vi "ROSNode.vi"(2 "Response":T1, 3 "ROS":T3={"topic port"=7000, "Node"="/LVROS", "topic"="/LVROS", "type"="", "node port"=7000, "error "={"status"=FALSE, "code"=0, "source"=""}, "Direction"=enum."Node", "Update (ms)"=1, "FIFO size"=1}) -> ()   [LabVIEW 2012]
doc: "Performs the functions of a ROS node: adds a publisher to the registered publisher list and registers with the master, starts and updates publishers, adds subscribers, and opens ports for subscribers and publishers"
uses:
  <userlib>/ROSforLV/ROS/Code/SubVIs/_ROSControl.ctl
  <userlib>/ROSforLV/ROS/Code/SubVIs/_ROSDirection.ctl
  <userlib>/ROSforLV/ROS/Code/Console/Servers/ServerSubs/MyState.ctl
  <userlib>/ROSforLV/ROS/Code/Console/Servers/ServerSubs/ROSLog.ctl
  <vilib>/Utility/miscctls.llb/LVPointTypeDef.ctl
  <userlib>/ROSforLV/ROS/Code/_ROSDefinition.vi
  <vilib>/Platform/browser.llb/Open URL in Default Browser (string).vi
panel:
  out "Color Code":picture
  out "Status out":T2[](array[typedef])
  out "Status":string
  out "Connections":bool
  out "Boundaries":cluster{i32, i32}[](array[cluster])=[{10, 22}, {30, 42}, {50, 62}]
  out "selection":i32=-1
  in  "HTML":bool
  out "ROS Master":string="130.64.16.138:11311"
  out "Registered":T3[](array[typedef])
  out "Last requestTopic":string
  out "Subscribers":T5(array[cluster])
  out "Queue log":string
  out "MyState":T2
  out "Setup":string
  in  "stop":bool
  out "HTML":picture
  out "Servers":picture
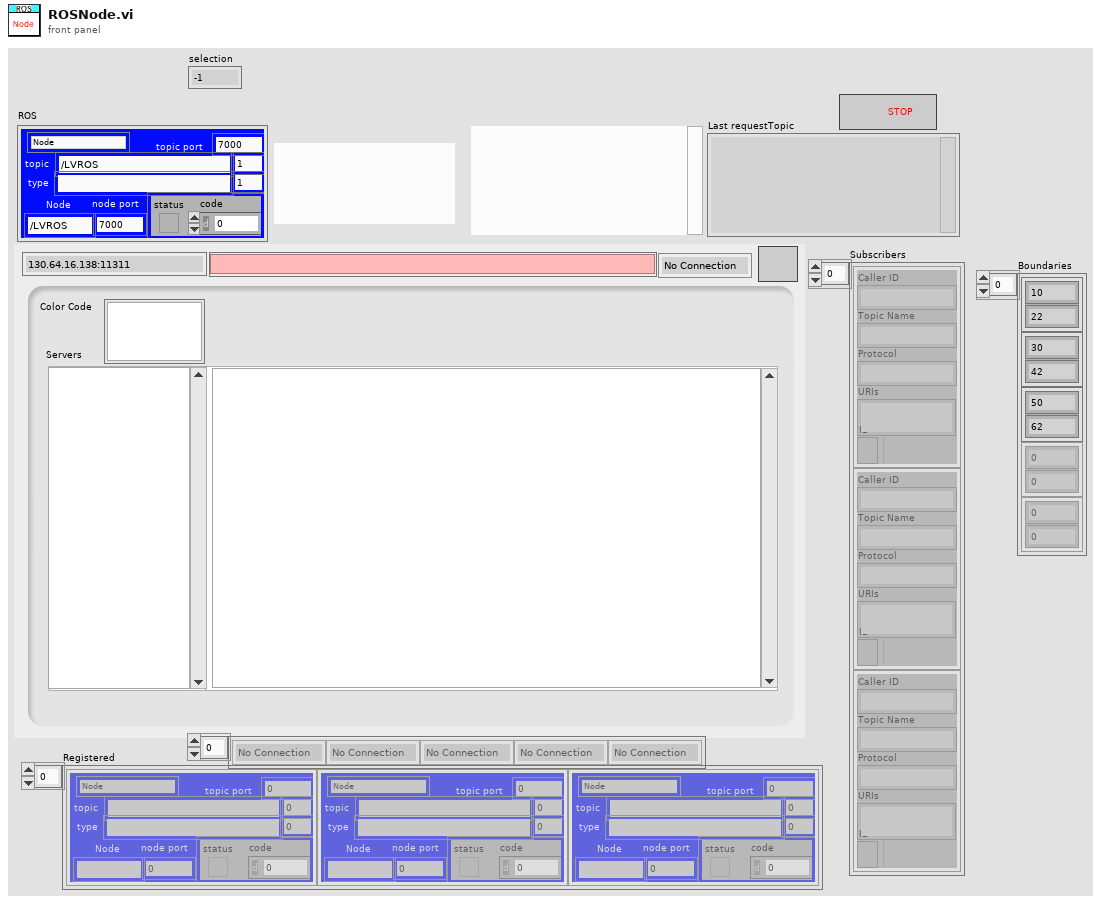
[diagram p1: front panel]
types:
  T1 = cluster{"Code":i32, "Status Message":string, "Nodes with this topic":string[]}
  T2 = typedef "MyState.ctl" = enum16{"No Connection", "Registered", "Connected", "Close"}
  T3 = typedef "_ROSControl.ctl" = cluster{"topic port":u16, "Node":string, "topic":string, "type":string, "node port":u16, "error ":errorcluster, "Direction":T4, "Update (ms)":u16, "FIFO size":u16}
  T4 = typedef "_ROSDirection.ctl" = enum16{"Node", "Publisher", "Subscriber", "ServiceClient", "ServiceProvider"}
  T5 = cluster{"Caller ID":string, "Topic Name":string, "Protocol":string, "URIs":string, "ID":refnum<k5>}[]
  T6 = enum16{"Reset Log", "Add Client", "Remove Client", "Add Task"}
  T7 = typedef "ROSLog.ctl" = cluster{"Sent":string, "Reply":string, "MethodName":string, "success":bool, "Dir1":string, "Dir2":string, "Time Stamp":string, "error":errorcluster, "Preamble":string, "Midamble":string, "Postamble":string}
  T8 = cluster{"Caller ID":string, "Topic Name":string, "Protocol":string, "URI":string, "ID":refnum<k5>}
  T9 = cluster{"Caller ID":string, "Topic Name":string, "Protocol":string, "URI":string, "ID":refnum<k5>}[]
  T10 = typedef "LVPointTypeDef.ctl" = cluster{"Horizontal":i16, "Vertical":i16}
  T11 = typedef "LVMouseTypeDef.ctl" = cluster{"Mouse Position":cluster{"X":i32, "Y":i32}, "Mouse Modifiers":cluster{"Button Down":bool, "Shift Mod":bool, "Menu Mod":bool, "Option Mod":bool}}
  T12 = cluster{"Caller ID":string, "Topic Name":string, "Node URIs":string[]}
  T13 = enum32{"Invalid", "Standard", "Closed", "Hidden", "Minimized", "Maximized"}
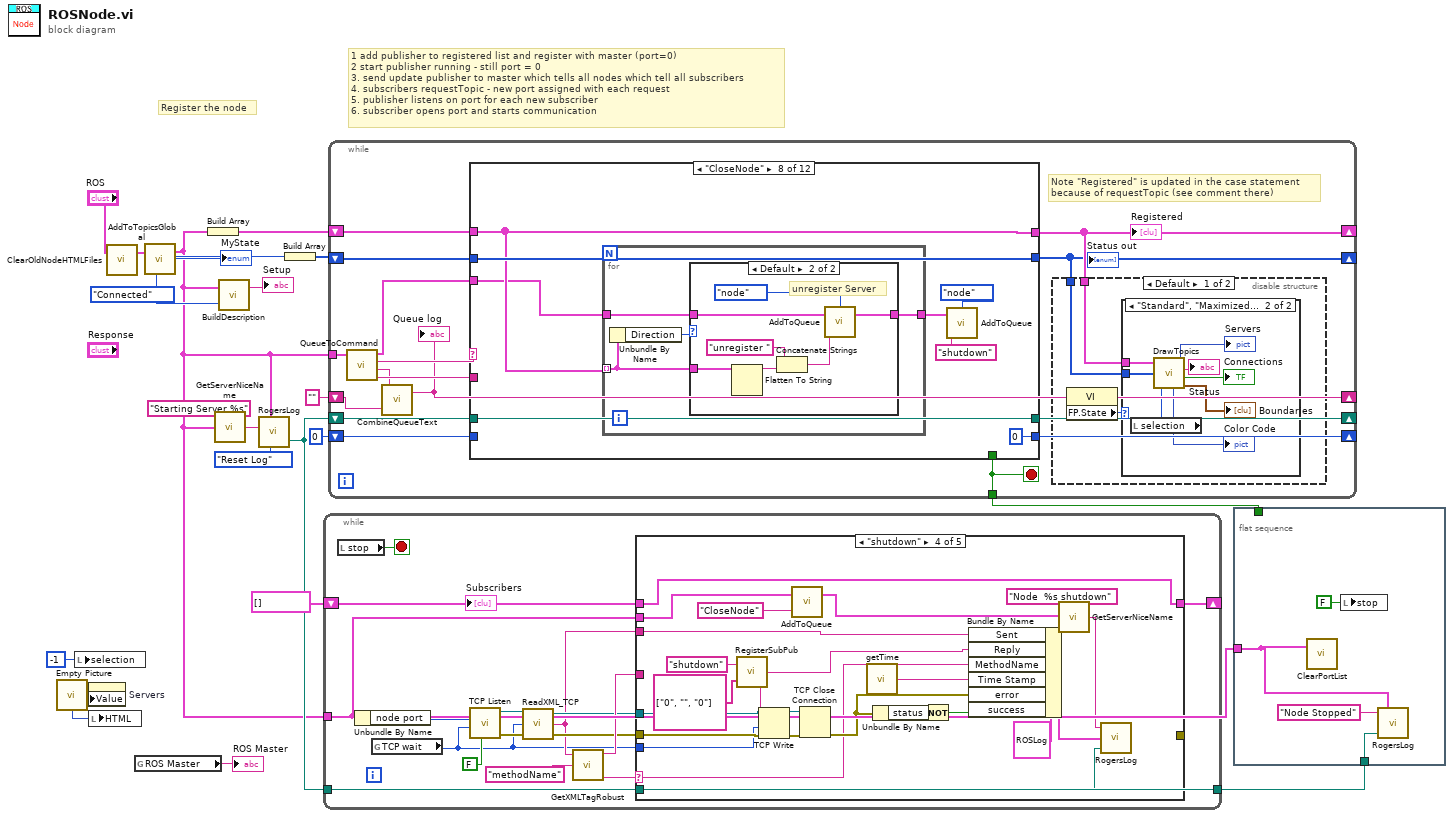
[diagram p0: block diagram]
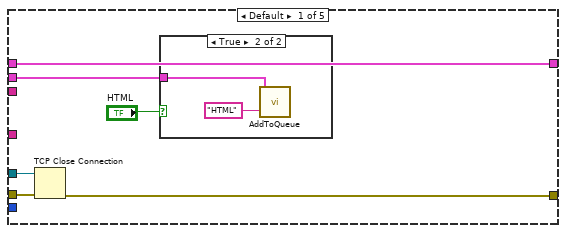
[diagram p2: hidden frame]
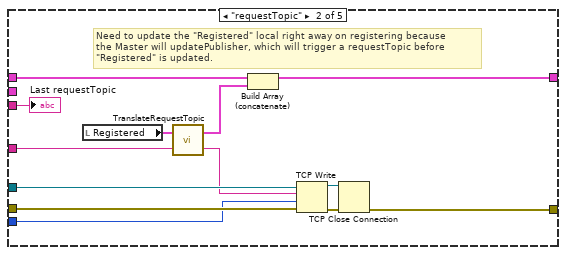
[diagram p4: hidden frame]
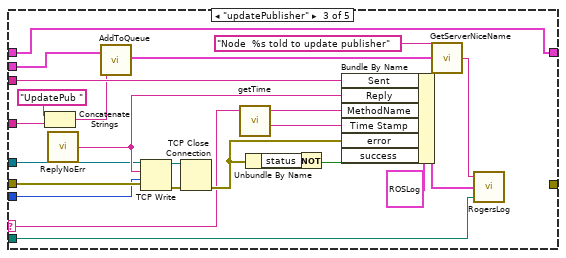
[diagram p5: hidden frame]
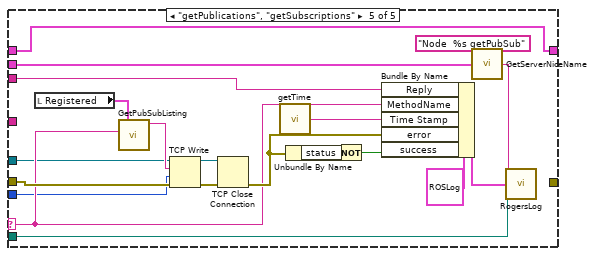
[diagram p6: hidden frame]
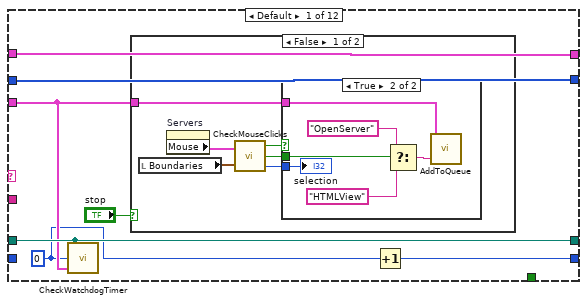
[diagram p9: hidden frame]
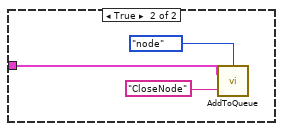
[diagram p11: hidden frame]
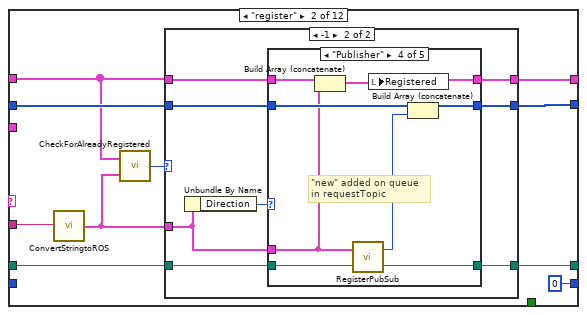
[diagram p12: hidden frame]
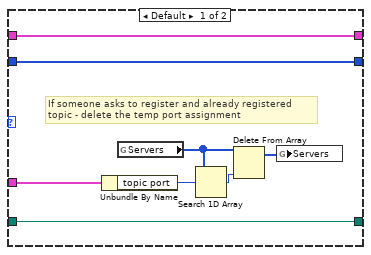
[diagram p13: hidden frame]
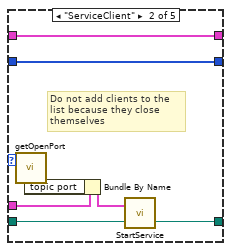
[diagram p15: hidden frame]
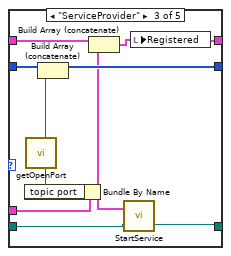
[diagram p16: hidden frame]
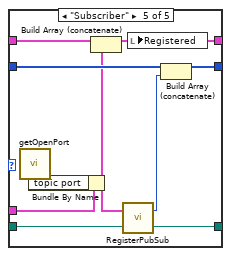
[diagram p17: hidden frame]
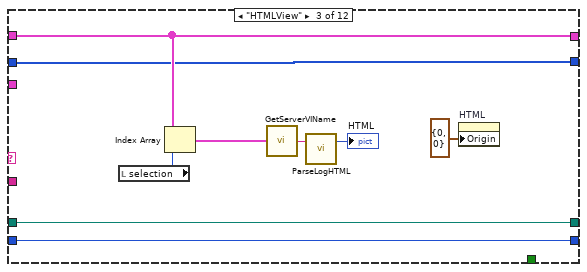
[diagram p18: hidden frame]
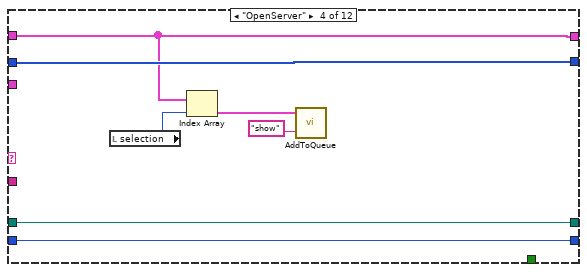
[diagram p19: hidden frame]
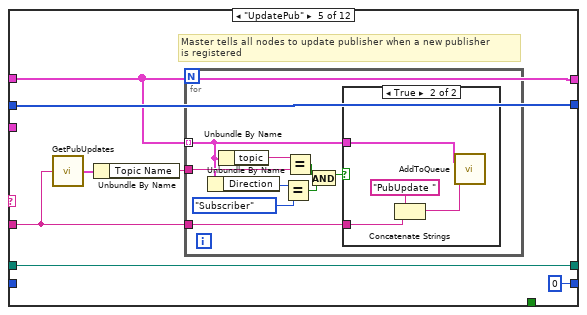
[diagram p20: hidden frame]
diagram:
  w12 = MyState."Connected" ("MyState")
  # "Register the node"
  # "1 add publisher to registered list and register with master (port=0)\n2 start publisher running - still port = 0\n3. send update publisher to master which tells all nodes which tell all subscribers\n4. subscribers requestTopic - new port assigned with each request\n5. publisher listens on port for each new subscriber\n6. subscriber opens port and starts communication"
  n1 = call "Empty Picture"() -> ("empty picture"=w10:picture)
  n2 = local write "selection"(-1 ("selection")) -> ()
  n3 = property on="Servers" class="Pict"("Value"=w10) -> ()  [unwired: 2 in, 2 out]
  n4 = local write "HTML"(w10) -> ()
  n5 = call <userlib>:"ClearOldNodeHTMLFiles.vi"("ROS"="ROS") -> ("ROS out"=w2:T3)  [unwired: 2 in]
  n6 = global read "_ROSDefinition.vi" "ROS Master"() -> (→"ROS Master":string)
  n7 = call <userlib>:"AddToTopicsGlobal.vi"("ROS in"=w2) -> ("ROS out"=w1:T3)  [unwired: 2 in]
  n8 = Build Array(w1) -> (w13:T3[])
  n9 = call <userlib>:"GetServerNiceName.vi"("ROS"=w1, "Text to add"="Starting Server %s") -> ("String"=w17:string)
  n10 = call <userlib>:"BuildDescription.vi"("MyState"=w12, "ROS in"=w1) -> ("Setup"=→"Setup":string)  [unwired: 1 in]
  n11 = call <userlib>:"RogersLog.vi"("Text to add"=w17, "ROS"=w1, "Task"=T6."Reset Log") -> ("LogPath out"=w7:path)  [unwired: 2 in, 1 out]
  n12 = Build Array(w12) -> (w11:T2[])
  n13 = while {
    shift-right: [w26] -> _
    shift-left: T5 [] ("Subscribers") -> [w27]
    tunnel: w1 -> [w21]
    tunnel: w7 -> [w20]
    tunnel: [w20] -> w4
    stop <- w35 stop-if-true
    n14 = local read "stop"() -> (w35:bool)
    n15 = Unbundle By Name(w21) -> ("node port"=w31:u16)
    n16 = global read "_ROSDefinition.vi" "TCP wait"() -> (w22:i32)
    n17 = call <vilib>:"TCP Listen.vi"("resolve remote address (T)"=FALSE, "timeout ms (wait forever: -1)"=w22, "port"=w31) -> ("error out"=w33:errorcluster, "connection ID"=w32:refnum<k5>)  [unwired: 4 in, 3 out]
    n18 = call <userlib>:"ReadXML_TCP.vi"("error in"=w33, "timeout ms (3000)"=w22, "connection ID in"=w32) -> ("error out"=w24:errorcluster, "data out"=w23:string, "connection ID out"=w25:refnum<k5>)
    n19 = call <userlib>:"GetXMLTagRobust.vi"("Tag"="methodName", "String"=w23) -> ("value"=w29:string, "String w/o Tag"=w28:string)  [unwired: 1 in, 2 out]
    n20 = case shown="\"shutdown\"" w29 {
      selector: w29 -> [_ _ w68 w97 w108]
      tunnel: w28 -> [_ w48 w65 _ _]
      tunnel: w27 -> [w41 w56 w66 w96 w115]
      tunnel: [w41 w55 w66 w96 w115] -> w26
      tunnel: w25 -> [w37 w52 w70 w86 w104]
      tunnel: w24 -> [w38 w51 w69 w88 w110]
      tunnel: w23 -> [_ w50 w71 w91 w116]
      tunnel: w22 -> [_ w45 w67 w83 w105]
      tunnel: w21 -> [w40 _ w57 w82 w109]
      tunnel: w20 -> [_ _ w60 w92 w111]
      tunnel: [w36 w44 _ _ _] -> _
      frame Default {
        n21 = TCP Close Connection(connection ID=w37, error in (no error)=w38) -> (error out=w36:errorcluster)  [unwired: 1 in, 1 out]
        n22 = case shown="True" "HTML" {
          tunnel: w40 -> [_ w42]
          frame False {
          }
          frame True {
            n23 = call <userlib>:"AddToQueue.vi"("Cmd"="HTML" ("element"), "ROS"=w42) -> ()  [unwired: 3 in, 1 out]
          }
        }
      }
      frame "requestTopic" {
        # "Need to update the \"Registered\" local right away on registering because\nthe Master will updatePublisher, which will trigger a requestTopic before\n\"Registered\" is updated."
        n24 = local read "Registered"() -> (w49:T3[])
        n25 = call <userlib>:"TranslateRequestTopic.vi"("String w/o Tag"=w48, "Registered"=w49) -> ("XML"=w47:string, "New Sub"=w46:T8)
        n26 = Build Array (concatenate)(w56, w46) -> (w55:T9)
        n27 = TCP Write(connection ID=w52, data in=w47, error in (no error)=w51, 9:w45) -> (connection ID out=w54:refnum<k5>, error out=w53:errorcluster)  [unwired: 1 out]
        n28 = TCP Close Connection(connection ID=w54, error in (no error)=w53) -> (error out=w44:errorcluster)  [unwired: 1 in, 1 out]
        "Last requestTopic" <- w50
      }
      frame "updatePublisher" {
        n29 = Concatenate Strings("UpdatePub " ("string"), w65) -> (w58:string)
        n30 = call <userlib>:"ReplyNoErr.vi"() -> ("msg out"=w75:string)  [unwired: 1 in]
        n31 = call <userlib>:"AddToQueue.vi"("Cmd"=w58, "ROS"=w57) -> ("ROS out"=w59:T3)  [unwired: 3 in]
        n32 = TCP Write(connection ID=w70, data in=w75, error in (no error)=w69, 9:w67) -> (connection ID out=w77:refnum<k5>, error out=w76:errorcluster)  [unwired: 1 out]
        n33 = TCP Close Connection(connection ID=w77, error in (no error)=w76) -> (error out=w74:errorcluster)  [unwired: 1 in, 1 out]
        n34 = call <userlib>:"getTime.vi"() -> ("Current Time"=w78:string)  [unwired: 1 in]
        n35 = Unbundle By Name(w74) -> ("status"=w73:bool)
        n36 = Not(x=w73) -> (.not. x?=w72:bool)
        n37 = Bundle By Name(cluster=T7 {"Sent"="", "Reply"="", "MethodName"="", "success"=TRUE, "Dir1"="From Master", "Dir2"="To Master", "Time Stamp"="", "error"={"status"=FALSE, "code"=0, "source"=""}, "Preamble"="", "Midamble"="", "Postamble"=""} ("Log"), "Sent"=w71, "Reply"=w75, "MethodName"=w68, "Time Stamp"=w78, "error"=w74, "success"=w72) -> (w63:T7)
        n38 = call <userlib>:"GetServerNiceName.vi"("ROS"=w59, "Text to add"="Node  %s told to update publisher") -> ("String"=w61:string)
        n39 = call <userlib>:"RogersLog.vi"("Text to add"=w61, "Log"=w63, "LogPath in"=w60) -> ()  [unwired: 2 in, 2 out]
      }
      frame "shutdown" {
        n40 = call <userlib>:"RegisterSubPub.vi"("Parameters"=string[] ["0", "", "0"], "MethodName"="shutdown") -> ("XML"=w85:string)
        n41 = TCP Write(connection ID=w86, data in=w85, error in (no error)=w88, 9:w83) -> (connection ID out=w84:refnum<k5>, error out=w87:errorcluster)  [unwired: 1 out]
        n42 = call <userlib>:"AddToQueue.vi"("Cmd"="CloseNode" ("element"), "ROS"=w82) -> ("ROS out"=w80:T3)  [unwired: 3 in]
        n43 = TCP Close Connection(connection ID=w84, error in (no error)=w87) -> (error out=w100:errorcluster)  [unwired: 1 in, 1 out]
        n44 = call <userlib>:"getTime.vi"() -> ("Current Time"=w101:string)  [unwired: 1 in]
        n45 = Unbundle By Name(w100) -> ("status"=w99:bool)
        n46 = Not(x=w99) -> (.not. x?=w98:bool)
        n47 = Bundle By Name(cluster=T7 {"Sent"="", "Reply"="", "MethodName"="", "success"=TRUE, "Dir1"="From Master", "Dir2"="To Master", "Time Stamp"="", "error"={"status"=FALSE, "code"=0, "source"=""}, "Preamble"="", "Midamble"="", "Postamble"=""} ("Log"), "Sent"=w91, "Reply"=w85, "MethodName"=w97, "Time Stamp"=w101, "error"=w100, "success"=w98) -> (w95:T7)
        n48 = call <userlib>:"GetServerNiceName.vi"("ROS"=w80, "Text to add"="Node  %s shutdown") -> ("String"=w93:string)
        n49 = call <userlib>:"RogersLog.vi"("Text to add"=w93, "Log"=w95, "LogPath in"=w92) -> ()  [unwired: 2 in, 2 out]
      }
      frame "getPublications", "getSubscriptions" {
        n50 = local read "Registered"() -> (w106:T3[])
        n51 = call <userlib>:"GetPubSubListing.vi"("Method"=w108, "Registered"=w106) -> ("StatusMessage"=w107:string)  [unwired: 9 in]
        n52 = TCP Write(connection ID=w104, data in=w107, 9:w105) -> (connection ID out=w103:refnum<k5>)  [unwired: 1 in, 2 out]
        n53 = TCP Close Connection(connection ID=w103, error in (no error)=w110) -> (error out=w119:errorcluster)  [unwired: 1 in, 1 out]
        n54 = call <userlib>:"getTime.vi"() -> ("Current Time"=w120:string)  [unwired: 1 in]
        n55 = Unbundle By Name(w119) -> ("status"=w118:bool)
        n56 = Not(x=w118) -> (.not. x?=w117:bool)
        n57 = Bundle By Name(cluster=T7 {"Sent"="", "Reply"="", "MethodName"="", "success"=TRUE, "Dir1"="From Master", "Dir2"="To Master", "Time Stamp"="", "error"={"status"=FALSE, "code"=0, "source"=""}, "Preamble"="", "Midamble"="", "Postamble"=""} ("Log"), "Reply"=w116, "MethodName"=w108, "Time Stamp"=w120, "error"=w119, "success"=w117) -> (w114:T7)
        n58 = call <userlib>:"GetServerNiceName.vi"("ROS"=w109, "Text to add"="Node  %s getPubSub") -> ("String"=w112:string)
        n59 = call <userlib>:"RogersLog.vi"("Text to add"=w112, "Log"=w114, "LogPath in"=w111) -> ()  [unwired: 2 in, 2 out]
      }
    }
    "Subscribers" <- w27
  }
  n60 = while {
    tunnel: w1 -> [w131]
    tunnel: [w134] -> w14
    shift-right: [w130] -> _
    shift-left: w13 -> [w135]
    shift-right: [w132] -> _
    shift-left: w7 -> [w133]
    shift-right: [w128] -> _
    shift-left: w11 -> [w129]
    shift-right: [w126] -> _
    shift-left: 0 ("selection") -> [w127]
    shift-right: [w125] -> _
    shift-left: "" ("New List") -> [w124]
    stop <- w134 stop-if-true
    # "Note \"Registered\" is updated in the case statement\nbecause of requestTopic (see comment there)"
    n61 = call <userlib>:"QueueToCommand.vi"("ROS"=w131) -> ("ROS out"=w122:T3, "Command"=w137:string, "Queue log"=w123:string, "data"=w136:string)  [unwired: 2 in]
    n62 = call <userlib>:"CombineQueueText.vi"("Old List"=w124, "Queue In"=w123) -> ("New List"=w125:string)  [unwired: 1 in]
    "Queue log" <- w125
    n63 = case shown="\"CloseNode\"" w137 {
      tunnel: w136 -> [_ w180 _ _ w251 w279 _ _ _ _ w337 _]
      tunnel: [w154 w179 w237 w247 w252 w273 w299 w307 w327 w331 w340 w357] -> w130
      tunnel: w135 -> [w154 w173 w237 w247 w252 w274 w300 w307 w327 w331 w340 w357]
      tunnel: [_ _ _ _ _ _ _ _ w324 _ _ _] -> w134
      tunnel: w133 -> [w152 w178 w239 w249 w256 w278 w302 w309 w325 w330 w346 w355]
      tunnel: [w152 w177 w239 w249 w256 w277 w302 w309 w325 w330 w346 w355] -> w132
      tunnel: w122 -> [w151 _ _ _ _ _ w294 w306 _ _ _ _]
      tunnel: w129 -> [w153 w176 w235 w248 w255 w272 w298 w310 w326 w329 w343 w356]
      tunnel: [w153 w175 w235 w248 w255 w271 w297 w310 w326 w329 w342 w356] -> w128
      tunnel: w127 -> [_ _ w234 w245 _ _ _ _ w323 w328 _ w354]
      tunnel: [w150 0 w234 w245 0 0 0 0 w323 w328 0 ("selection") w354] -> w126
      frame Default {
        w149 = 0 ("selection")
        n64 = call <userlib>:"CheckWatchdogTimer.vi"("ROS"=w151, "itteration"=w149, "LogPath in"=w152) -> ()  [unwired: 3 in]
        n65 = case shown="False" "stop" {
          tunnel: w151 -> [w158 w169]
          frame False {
            n66 = local read "Boundaries"() -> (w157:cluster{i32, i32}[])
            n67 = property on="Servers" class="Pict"() -> ("Mouse"=w159:T11)  [unwired: 2 in, 2 out]
            n68 = call <userlib>:"CheckMouseClicks.vi"("Mouse"=w159, "Boundaries"=w157) -> ("Change?"=w160:bool, "Shift?"=w156:bool, "selection"=w161:i32)
            n69 = case shown="True" w160 {
              tunnel: w161 -> [_ w167]
              tunnel: w158 -> [_ w162]
              tunnel: w156 -> [_ w165]
              frame False {
              }
              frame True {
                n70 = Select(t="OpenServer" ("element"), s=w165, f="HTMLView" ("element")) -> (s? t:f=w163:string)
                n71 = call <userlib>:"AddToQueue.vi"("Cmd"=w163, "ROS"=w162) -> ()  [unwired: 3 in, 1 out]
                "selection" <- w167
              }
            }
          }
          frame True {
            n72 = call <userlib>:"AddToQueue.vi"("Cmd"="CloseNode" ("element"), "ROS"=w169, "Type"=enum16{"topic", "node"}."node" ("Name")) -> ()  [unwired: 2 in, 1 out]
          }
        }
        n73 = Increment(x=w149) -> (x+1=w150:i32)
      }
      frame "register" {
        n74 = call <userlib>:"ConvertStringtoROS.vi"("string in"=w180) -> ("ROS"=w172:T3)
        n75 = call <userlib>:"CheckForAlreadyRegistered.vi"("ROS"=w172, "Registered"=w173) -> ("index of element"=w174:i32)
        n76 = case shown="-1" w174 {
          tunnel: w172 -> [w185 w189]
          tunnel: [w188 w196] -> w179
          tunnel: w173 -> [w188 w195]
          tunnel: w178 -> [w186 w194]
          tunnel: [w186 w193] -> w177
          tunnel: w176 -> [w187 w192]
          tunnel: [w187 w191] -> w175
          frame Default {
            # "If someone asks to register and already registered\ntopic - delete the temp port assignment"
            n77 = Unbundle By Name(w185) -> ("topic port"=w184:u16)
            n78 = global read "_ROSDefinition.vi" "Servers"() -> (w182:u16[])
            n79 = Search 1D Array(1D array=w182, element=w184) -> (index of element=w183:i32)  [unwired: 1 in]
            n80 = Delete From Array(array=w182, index=w183) -> (array with subset deleted=w181:u16[])  [unwired: 1 in, 1 out]
            n81 = global write "_ROSDefinition.vi" "Servers"(w181) -> ()
          }
          frame -1 {
            n82 = Unbundle By Name(w189) -> ("Direction"=w190:T4)
            n83 = case shown="\"Publisher\"" w190 {
              tunnel: [w199 w201 w212 w216 w224] -> w196
              tunnel: w195 -> [w199 w201 w214 w223 w233]
              tunnel: w194 -> [w197 w206 w208 w222 w232]
              tunnel: [w197 w205 w207 w221 w231] -> w193
              tunnel: w192 -> [w198 w200 w213 w220 w230]
              tunnel: [w198 w200 w211 w219 w229] -> w191
              tunnel: w189 -> [_ w203 w215 w217 w226]
              frame "Node", Default {
              }
              frame "ServiceClient" {
                # "Do not add clients to the \nlist because they close \nthemselves"
                n84 = call <userlib>:"getOpenPort.vi"() -> ("port"=w204:u16)
                n85 = Bundle By Name(cluster=w203, "topic port"=w204) -> (w202:T3)
                n86 = call <userlib>:"StartService.vi"("LogPath in"=w206, "New server ROS"=w202) -> ("LogPath out"=w205:path)  [unwired: 1 out]
              }
              frame "ServiceProvider" {
                n87 = call <userlib>:"getOpenPort.vi"() -> ("port"=w210:u16)
                n88 = Bundle By Name(cluster=w215, "topic port"=w210) -> (w209:T3)
                n89 = Build Array (concatenate)(w213, w210) -> (w211:u16[])
                n90 = Build Array (concatenate)(w214, w209) -> (w212:T3[])
                n91 = call <userlib>:"StartService.vi"("LogPath in"=w208, "New server ROS"=w209) -> ("LogPath out"=w207:path)  [unwired: 1 out]
                n92 = local write "Registered"(w212) -> ()
              }
              frame "Publisher" {
                # "\"new\" added on queue\nin requestTopic"
                n93 = Build Array (concatenate)(w223, w217) -> (w216:T3[])
                n94 = call <userlib>:"RegisterPubSub.vi"("LogPath in"=w222, "New server ROS"=w217) -> ("LogPath out"=w221:path, "MyState"=w218:T2)
                n95 = local write "Registered"(w216) -> ()
                n96 = Build Array (concatenate)(w220, w218) -> (w219:u16[])
              }
              frame "Subscriber" {
                n97 = call <userlib>:"getOpenPort.vi"() -> ("port"=w227:u16)
                n98 = Bundle By Name(cluster=w226, "topic port"=w227) -> (w225:T3)
                n99 = Build Array (concatenate)(w233, w225) -> (w224:T3[])
                n100 = call <userlib>:"RegisterPubSub.vi"("LogPath in"=w232, "New server ROS"=w225) -> ("LogPath out"=w231:path, "MyState"=w228:T2)
                n101 = local write "Registered"(w224) -> ()
                n102 = Build Array (concatenate)(w230, w228) -> (w229:u16[])
              }
            }
          }
        }
      }
      frame "HTMLView" {
        n103 = local read "selection"() -> (w240:i32)
        n104 = Index Array(array=w237, index=w240) -> (element=w236:T3)
        n105 = call <userlib>:"GetServerVIName.vi"("ROS"=w236) -> ("vi name"=w241:string)
        n106 = call <userlib>:"ParseLogHTML.vi"("vi name"=w241) -> ("2D Picture"=→"HTML":picture)  [unwired: 1 in, 1 out]
        n107 = property on="HTML" class="Pict"("Origin"=T10 {"Horizontal"=0, "Vertical"=0}) -> ()  [unwired: 2 in, 2 out]
      }
      frame "OpenServer" {
        n108 = local read "selection"() -> (w246:i32)
        n109 = Index Array(array=w247, index=w246) -> (element=w244:T3)
        n110 = call <userlib>:"AddToQueue.vi"("Cmd"="show" ("element"), "ROS"=w244) -> ()  [unwired: 3 in, 1 out]
      }
      frame "UpdatePub" {
        # "Master tells all nodes to update publisher when a new publisher\nis registered"
        n111 = call <userlib>:"GetPubUpdates.vi"("XML"=w251) -> ("PubUpdate"=w254:T12)
        n112 = Unbundle By Name(w254) -> ("Topic Name"=w253:string)
        n113 = for {
          tunnel: w252 -> [w258] mode=indexing
          tunnel: w253 -> [w264]
          tunnel: w251 -> [w257]
          n114 = Unbundle By Name(w258) -> ("Direction"=w263:T4)
          n115 = Unbundle By Name(w258) -> ("topic"=w265:string)
          n116 = Equal?(x=w263, y=_ROSDirection."Subscriber" ("Direction")) -> (x = y?=w260:bool)
          n117 = Equal?(x=w265, y=w264) -> (x = y?=w261:bool)
          n118 = And(x=w261, y=w260) -> (x .and. y?=w259:bool)
          n119 = case shown="True" w259 {
            tunnel: w258 -> [_ w266]
            tunnel: w257 -> [_ w268]
            frame False {
            }
            frame True {
              n120 = Concatenate Strings("PubUpdate " ("string"), w268) -> (w267:string)
              n121 = call <userlib>:"AddToQueue.vi"("Cmd"=w267, "ROS"=w266) -> ()  [unwired: 3 in, 1 out]
            }
          }
        }
      }
      frame "unregister" {
        n122 = call <userlib>:"ConvertStringtoROS.vi"("string in"=w279) -> ("ROS"=w276:T3)
        n123 = call <userlib>:"CheckForAlreadyRegistered.vi"("ROS"=w276, "Registered"=w274) -> ("index of element"=w275:i32)
        n124 = case shown="Default" w275 {
          selector: w275 -> [_ w286]
          tunnel: w278 -> [w280 w292]
          tunnel: [w280 w291] -> w277
          tunnel: w276 -> [_ w284]
          tunnel: w274 -> [w282 w285]
          tunnel: [w282 w289] -> w273
          tunnel: w272 -> [w281 w288]
          tunnel: [w281 w287] -> w271
          frame -1 {
          }
          frame Default {
            # "Stop Server"
            n125 = Delete From Array(array=w285, index=w286) -> (array with subset deleted=w289:T3[])  [unwired: 1 in, 1 out]
            n126 = Delete From Array(array=w288, index=w286) -> (array with subset deleted=w287:u16[])  [unwired: 1 in, 1 out]
            n127 = call <userlib>:"UnRegisterPubSub.vi"("LogPath in"=w292, "ROS"=w284) -> ("LogPath out"=w291:path)  [unwired: 1 out]
            n128 = call <userlib>:"AddToQueue.vi"("Cmd"="done" ("element"), "ROS"=w284, "Type"=enum16{"topic", "node"}."topic" ("Name")) -> ()  [unwired: 2 in, 1 out]
          }
        }
      }
      frame "shutdown" {
        # "Stop Server"
        n129 = call <userlib>:"CheckForAlreadyRegistered.vi"("ROS"=w294, "Registered"=w300) -> ("index of element"=w301:i32)
        n130 = call <userlib>:"AddToQueue.vi"("Cmd"="done" ("element"), "ROS"=w294, "Type"=enum16{"topic", "node"}."node" ("Name")) -> ()  [unwired: 2 in, 1 out]
        n131 = Delete From Array(array=w300, index=w301) -> (array with subset deleted=w299:T3[])  [unwired: 1 in, 1 out]
        n132 = Delete From Array(array=w298, index=w301) -> (array with subset deleted=w297:u16[])  [unwired: 1 in, 1 out]
      }
      frame "CloseNode" {
        n133 = for {
          tunnel: w307 -> [w314] mode=indexing
          tunnel: w306 -> [w312]
          tunnel: [w311] -> w304
          n134 = Unbundle By Name(w314) -> ("Direction"=w313:T4)
          n135 = case shown="Default" w313 {
            tunnel: w314 -> [_ w322]
            tunnel: w312 -> [w315 w319]
            tunnel: [w315 w316] -> w311
            frame "Node" {
              # "Provider closes in server\nand Node closes in \nshutdown."
            }
            frame Default {
              # "unregister Server"
              n136 = Flatten To String(anything=w322) -> (data string=w321:string)  [unwired: 3 in, 2 out]
              n137 = Concatenate Strings("unregister " ("element"), w321) -> (w318:string)
              n138 = call <userlib>:"AddToQueue.vi"("Cmd"=w318, "ROS"=w319, "Type"=enum16{"topic", "node"}."node" ("Name")) -> ("ROS out"=w316:T3)  [unwired: 2 in]
            }
          }
        }
        n139 = call <userlib>:"AddToQueue.vi"("Cmd"="shutdown" ("element"), "ROS"=w304, "Type"=enum16{"topic", "node"}."node" ("Name")) -> ()  [unwired: 2 in, 1 out]
      }
      frame "done" {
        w324 = TRUE ("stop")
        n140 = local write "stop"(w324) -> ()
      }
      frame "HTML" {
        n141 = disable-structure shown="Default" {
          disable-tunnel: w330 -> [w332 _]
          frame condition #0 (active) {
            n142 = call <userlib>:"GetLogFilePath.vi"() -> ("LogFolder"=w334:path)  [unwired: 2 in, 1 out]
            n143 = Build Path(base path=w334, name or relative path="index.html" ("pattern")) -> ()  [unwired: 1 out]
            n144 = call <vilib>:"Path to URL.vi"("path"=w332) -> ("url"=w335:string)
            n145 = call-poly <vilib>:"Open URL in Default Browser.vi"("URL"=w335) -> ()  [unwired: 5 in, 2 out]
          }
          frame condition #1 {
          }
        }
      }
      frame "status" {
        n146 = Match Pattern(string=w337, regular expression="STATE") -> (before substring=w341:string, after substring=w344:string)  [unwired: 1 in, 2 out]
        n147 = call <userlib>:"ConvertStringtoROS.vi"("string in"=w341) -> ("ROS"=w339:T3)
        n148 = call <userlib>:"CheckForAlreadyRegistered.vi"("ROS"=w339, "Registered"=w340) -> ("index of element"=w338:i32)
        n149 = case shown="Default" w338 {
          selector: w338 -> [w350 _]
          tunnel: w344 -> [w352 _]
          tunnel: w343 -> [w351 w353]
          tunnel: [w348 w353] -> w342
          frame Default {
            n150 = Scan From String(format string="%d", input string=w352) -> (output 1=w349:i32)  [unwired: 3 in, 3 out]
            n151 = Replace Array Subset(array=w351, new element=w349, index=w350) -> (w348:u16[])
          }
          frame -1 {
          }
        }
      }
      frame "show" {
        n152 = control-ref of="This VI"() -> (w358:refnum<vi>)
        n153 = invoke class="VI" method="FP.Open"(reference=w358) -> ()  [unwired: 4 in, 5 out]
      }
    }
    "Registered" <- w130
    "Status out" <- w128
    n154 = disable-structure shown="Default" {
      disable-tunnel: w130 -> [w140 _]
      disable-tunnel: w128 -> [w139 _]
      frame condition #0 (active) {
        n155 = property class="VI"() -> ("FP.State"=w138:T13)  [unwired: 2 in, 2 out]
        n156 = case shown="\"Standard\", \"Maximized\"" w138 {
          tunnel: w140 -> [_ w143]
          tunnel: w139 -> [_ w142]
          frame "Invalid", Default {
          }
          frame "Standard", "Maximized" {
            n157 = local read "selection"() -> (w147:i32)
            n158 = call <userlib>:"DrawTopics.vi"("Registered"=w143, "Status"=w142, "Selection"=w147) -> ("new picture"=→"Servers":picture, "Status"=→"Status":string, "all good?"=→"Connections":bool, "Boundaries"=→"Boundaries":cluster{i32, i32}[], "Key"=→"Color Code":picture)
          }
        }
      }
      frame condition #1 {
      }
    }
  }
  n159 = flat-sequence {
    tunnel: w14 -> [_]
    tunnel: w4 -> [w360]
    tunnel: w1 -> [w359]
    frame #0 {
      n160 = call <userlib>:"ClearPortList.vi"("ROS"=w359) -> ()  [unwired: 2 in]
      n161 = local write "stop"(FALSE ("stop")) -> ()
      n162 = call <userlib>:"RogersLog.vi"("Text to add"="Node Stopped", "ROS"=w359, "LogPath in"=w360) -> ()  [unwired: 2 in, 2 out]
    }
  }
  "MyState" <- w12
